vi "Teleop.vi"(10 "Match Info":T1={"Autonomous Elapsed Seconds"=0.0, "TeleOp Elapsed Seconds"=0.0, "Disabled Elapsed Seconds"=0.0, "Visited Autonomous"=FALSE, "Visited TeleOp"=FALSE, "Visited Disabled"=FALSE, "Autonomous Settings"={"Autonomous Style"=enum."Independent", "VI Refnum"=refnum}}, 11 "Call Context":T2) -> ()   [LabVIEW 2020]
doc: "This VI is called for each TeleOp packet received from the DS where the robot is not disabled. It is often used to read from the joysticks and update I/O or to update setpoints for timed control loops. It should complete and return within 20 milliseconds or it may miss DS packets."
uses:
  <vilib>/Rock Robotics/WPI/DriverStation/WPI_DriverStationDerivedRobotMode.ctl
  <vilib>/Rock Robotics/WPI/DriverStation/WPI_DriverStationMatch Info.ctl
  <vilib>/Rock Robotics/WPI/Utilities/WPI_GetSetVariantRefNum.vi
  Robot Global Data.vi
  <vilib>/Rock Robotics/Network Tables/NT Write Boolean Array.vi
  <vilib>/Rock Robotics/Network Tables/NT Write Numeric Array.vi
  <vilib>/Rock Robotics/Network Tables/NT Read Boolean.vi
  SUB VIs/TOGGLE GLOBAL.vi
  <vilib>/Rock Robotics/Network Tables/NT Read Number.vi
panel:
  out "Sample Slider 0":dbl(slide) scale=0.0..5.0
  out "Sample Boolean 1":bool
  out "Sample Boolean 0":bool
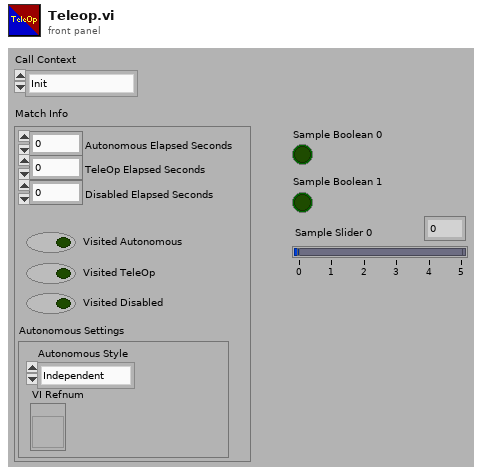
[diagram p1: front panel]
types:
  T1 = typedef "WPI_DriverStationMatch Info.ctl" = cluster{"Autonomous Elapsed Seconds":dbl, "TeleOp Elapsed Seconds":dbl, "Disabled Elapsed Seconds":dbl, "Visited Autonomous":bool, "Visited TeleOp":bool, "Visited Disabled":bool, "Autonomous Settings":cluster{"Autonomous Style":enum16{"Iterative", "Independent"}, "VI Refnum":refnum<vi>}}
  T2 = typedef "WPI_DriverStationDerivedRobotMode.ctl" = enum16{"Init", "Execute", "Stop"}
  T3 = typedef "WPI_JoystickDevRef.ctl" = cluster{"Device":T4}
  T4 = typedef "WPI_JoystickDeviceEnum.ctl" = enum16{"USB 0", "USB 1", "USB 2", "USB 3", "USB 4", "USB 5"}
  T5 = cluster{"POVs[0]":i16, "POVs[1]":i16, "POVs[2]":i16, "POVs[3]":i16, "POVs[4]":i16, "POVs[5]":i16, "POVs[6]":i16, "POVs[7]":i16, "POVs[8]":i16}
  T6 = cluster{"Axes[0]":dbl, "Axes[1]":dbl, "Axes[2]":dbl, "Axes[3]":dbl, "Axes[4]":dbl, "Axes[5]":dbl, "Axes[6]":dbl, "Axes[7]":dbl, "Axes[8]":dbl}
  T7 = cluster{"Buttons[0]":bool, "Buttons[1]":bool, "Buttons[2]":bool, "Buttons[3]":bool, "Buttons[4]":bool, "Buttons[5]":bool, "Buttons[6]":bool, "Buttons[7]":bool, "Buttons[8]":bool}
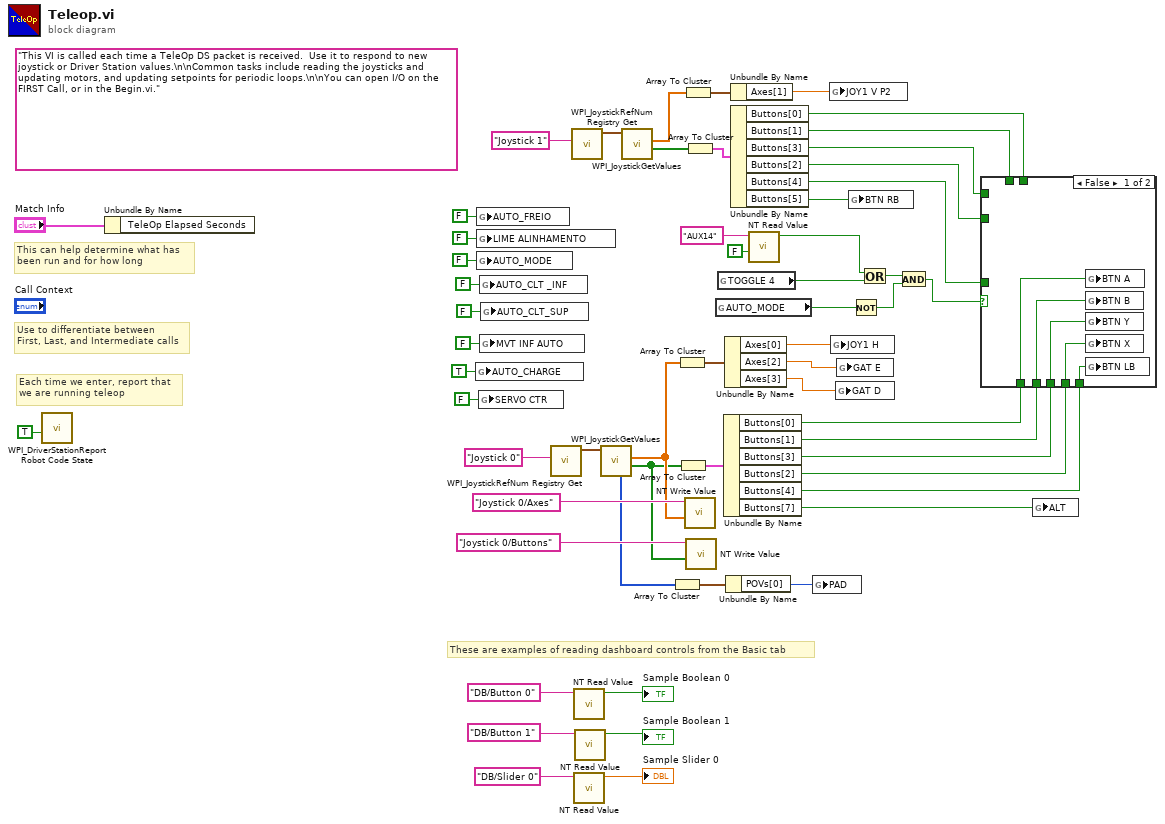
[diagram p0: block diagram]
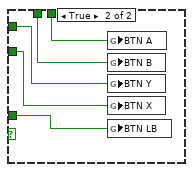
[diagram p2: hidden frame]
diagram:
  (unwired) "This VI is called each time a TeleOp DS packet is received.  Use it to respond to new joystick or Driver Station values.\n\nCommon tasks include reading the joysticks and updating motors, and updating setpoints for periodic loops.\n\nYou can open I/O on the FIRST Call, or in the Begin.vi."
  # "These are examples of reading dashboard controls from the Basic tab"
  # "Each time we enter, report that\nwe are running teleop"
  # "Use to differentiate between\nFirst, Last, and Intermediate calls"
  # "This can help determine what has\nbeen run and for how long"
  n1 = call <vilib>:"WPI_DriverStationReport Robot Code State.vi"("TeleOp"=TRUE ("Autonomous")) -> ()  [unwired: 10 in, 1 out]
  n2 = Unbundle By Name("Match Info") -> ()  [unwired: 1 out]
  n3 = global write "Robot Global Data.vi" "AUTO_CHARGE"(TRUE ("AUTO_CHARGE")) -> ()
  n4 = global write "Robot Global Data.vi" "AUTO_FREIO"(FALSE ("AUTO_FREIO")) -> ()
  n5 = global write "Robot Global Data.vi" "LIME ALINHAMENTO"(FALSE ("LIME ALINHAMENTO")) -> ()
  n6 = global write "Robot Global Data.vi" "AUTO_MODE"(FALSE ("AUTO_MODE")) -> ()
  n7 = global write "Robot Global Data.vi" "SERVO CTR"(FALSE ("SERVO CTR")) -> ()
  n8 = global write "Robot Global Data.vi" "AUTO_CLT _INF"(FALSE ("AUTO_CLT")) -> ()
  n9 = global write "Robot Global Data.vi" "MVT INF AUTO"(FALSE ("MVT INF AUTO")) -> ()
  n10 = global write "Robot Global Data.vi" "AUTO_CLT_SUP"(FALSE ("AUTO_CLT")) -> ()
  n11 = call <vilib>:"WPI_JoystickRefNum Registry Get.vi"("refnum name"="Joystick 0") -> ("JoystickDevRef"=w55:T3)  [unwired: 1 in, 9 out]
  n12 = call <vilib>:"WPI_JoystickRefNum Registry Get.vi"("refnum name"="Joystick 1") -> ("JoystickDevRef"=w38:T3)  [unwired: 1 in, 9 out]
  n13 = call-poly <vilib>:"NT Read Value.vi"("name"="DB/Button 0" ("refnum name")) -> ("value"=→"Sample Boolean 0":bool)  [unwired: 8 in, 2 out]
  n14 = call-poly <vilib>:"NT Read Value.vi"("name"="DB/Slider 0" ("refnum name")) -> ("value"=→"Sample Slider 0":dbl)  [unwired: 8 in, 2 out]
  n15 = call-poly <vilib>:"NT Read Value.vi"("name"="DB/Button 1" ("refnum name")) -> ("value"=→"Sample Boolean 1":bool)  [unwired: 8 in, 2 out]
  n16 = call <vilib>:"WPI_JoystickGetValues.vi"("JoystickDevRef"=w55) -> ("Buttons"=w42:bool[], "Axes"=w45:dbl[], "POVs"=w14:i16[])  [unwired: 6 in, 2 out]
  n17 = call <vilib>:"WPI_JoystickGetValues.vi"("JoystickDevRef"=w38) -> ("Buttons"=w32:bool[], "Axes"=w34:dbl[])  [unwired: 6 in, 3 out]
  n18 = Array To Cluster(array=w14) -> (cluster=w15:T5)
  n19 = Array To Cluster(array=w45) -> (cluster=w44:T6)
  n20 = Array To Cluster(array=w42) -> (cluster=w43:T7)
  n21 = Array To Cluster(array=w34) -> (cluster=w35:T6)
  n22 = Array To Cluster(array=w32) -> (cluster=w33:T7)
  n23 = call-poly <vilib>:"NT Write Value.vi"("value"=w45, "name"="Joystick 0/Axes" ("Name")) -> ()  [unwired: 9 in, 1 out]
  n24 = call-poly <vilib>:"NT Write Value.vi"("value"=w42, "name"="Joystick 0/Buttons" ("Name")) -> ()  [unwired: 9 in, 1 out]
  n25 = global read "Robot Global Data.vi" "AUTO_MODE"() -> (w5:bool)
  n26 = global read "TOGGLE GLOBAL.vi" "TOGGLE 4"() -> (w10:bool)
  n27 = Unbundle By Name(w43) -> ("Buttons[0]"=w20:bool, "Buttons[1]"=w21:bool, "Buttons[3]"=w22:bool, "Buttons[2]"=w23:bool, "Buttons[4]"=w24:bool, "Buttons[7]"=w12:bool)
  n28 = Unbundle By Name(w44) -> ("Axes[0]"=w41:dbl, "Axes[2]"=w40:dbl, "Axes[3]"=w39:dbl)
  n29 = Unbundle By Name(w15) -> ("POVs[0]"=w13:i16)
  n30 = Unbundle By Name(w35) -> ("Axes[1]"=w36:dbl)
  n31 = Unbundle By Name(w33) -> ("Buttons[0]"=w29:bool, "Buttons[1]"=w28:bool, "Buttons[3]"=w27:bool, "Buttons[2]"=w26:bool, "Buttons[4]"=w25:bool, "Buttons[5]"=w1:bool)
  n32 = call-poly <vilib>:"NT Read Value.vi"("default value"=FALSE, "name"="AUX14") -> ("value"=w11:bool)  [unwired: 7 in, 2 out]
  n33 = global write "Robot Global Data.vi" "PAD"(w13) -> ()
  n34 = global write "Robot Global Data.vi" "JOY1 V P2"(w36) -> ()
  n35 = global write "Robot Global Data.vi" "JOY1 H"(w41) -> ()
  n36 = global write "Robot Global Data.vi" "GAT D"(w39) -> ()
  n37 = global write "Robot Global Data.vi" "GAT E"(w40) -> ()
  n38 = global write "Robot Global Data.vi" "BTN RB"(w1) -> ()
  n39 = Not(x=w5) -> (.not. x?=w4:bool)
  n40 = Or(x=w11, y=w10) -> (x .or. y?=w7:bool)
  n41 = And(x=w7, y=w4) -> (x .and. y?=w6:bool)
  n42 = case shown="False" w6 {
    tunnel: w29 -> [_ w67]
    tunnel: w28 -> [_ w66]
    tunnel: w27 -> [_ w65]
    tunnel: w26 -> [_ w64]
    tunnel: w25 -> [_ w63]
    tunnel: w24 -> [w62 _]
    tunnel: w23 -> [w61 _]
    tunnel: w22 -> [w60 _]
    tunnel: w21 -> [w59 _]
    tunnel: w20 -> [w58 _]
    frame False {
      n43 = global write "Robot Global Data.vi" "BTN A"(w58) -> ()
      n44 = global write "Robot Global Data.vi" "BTN B"(w59) -> ()
      n45 = global write "Robot Global Data.vi" "BTN Y"(w60) -> ()
      n46 = global write "Robot Global Data.vi" "BTN X"(w61) -> ()
      n47 = global write "Robot Global Data.vi" "BTN LB"(w62) -> ()
    }
    frame True {
      n48 = global write "Robot Global Data.vi" "BTN A"(w67) -> ()
      n49 = global write "Robot Global Data.vi" "BTN B"(w66) -> ()
      n50 = global write "Robot Global Data.vi" "BTN Y"(w65) -> ()
      n51 = global write "Robot Global Data.vi" "BTN X"(w64) -> ()
      n52 = global write "Robot Global Data.vi" "BTN LB"(w63) -> ()
    }
  }
  n53 = global write "Robot Global Data.vi" "ALT"(w12) -> ()
